vi "Off.vi"(0 "reference in":refnum<class "Spindle.lvclass">, 5 "error in (no error)":errorcluster) -> (14 "reference out":refnum<class "Spindle.lvclass">, 19 "error out":errorcluster)   [LabVIEW 2013, in "Spindle.lvclass"]
uses:
  Spindle.lvclass
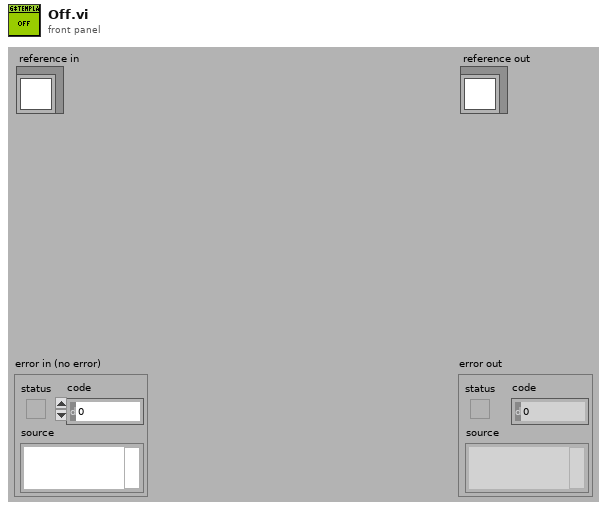
[diagram p1: front panel]
types:
  T1 = typedef "Spindle.lvclass/ObjectAttributes.ctl" = cluster{"Name":string}
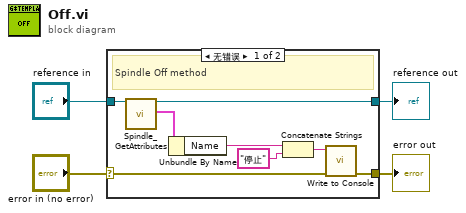
[diagram p0: block diagram]
diagram:
  n1 = case shown="无错误" "error in (no error)" {
    selector: "error in (no error)" -> [w6 w14]
    tunnel: [w5 w14] -> w3
    tunnel: [w7 w13] -> w1
    tunnel: "reference in" -> [w8 w13]
    frame No Error {
      # "Spindle Off method"
      n2 = call "Spindle_GetAttributes.vi"("reference in"=w8) -> ("reference out"=w7:refnum<class "Spindle.lvclass">, "attributes"=w9:T1)  [unwired: 15 in, 2 out]
      n3 = Unbundle By Name(w9) -> ("Name"=w10:string)
      n4 = Concatenate Strings(w10, "停止" ("Input")) -> (w12:string)
      n5 = call "Write to Console.vi"("error in (no error)"=w6, "Input"=w12) -> ("error out"=w5:errorcluster)  [unwired: 9 in]
    }
    frame Error {
    }
  }
  "error out" <- w3
  "reference out" <- w1
